vi "H5Pget_fill_value.vi"(4 "Data type":variant, 5 "HDF5 Type Ref (match data)":T1, 6 "error in (no error)":errorcluster, 9 "HDF5 Property Ref":T1) -> (0 "error out":errorcluster, 1 "Data Element":variant, 3 "HDF5 Ref out":T1)   [LabVIEW 2017]
doc: "Retrieves a dataset fill value."
uses:
  <vilib>/UPVI/lvhdf5/library.llb/HDF5 Ref.ctl
  <vilib>/UPVI/lvhdf5/identifier.llb/H5Iget_type.vi
  <vilib>/UPVI/lvhdf5/h5helper.dll
panel:
  # "LVHDF5 Toolkit\nCopyright (c) 2005-2013 by Jason D. Sommerville\nCopyright (c) 2014 by UPVI, LLC.\n\nThis use and distribution of this file is governed by the terms found in \nLICENSE.txt distributed with this toolkit and installed at\n <user.lib>\\_lvhdf5\\LICENSE.txt"
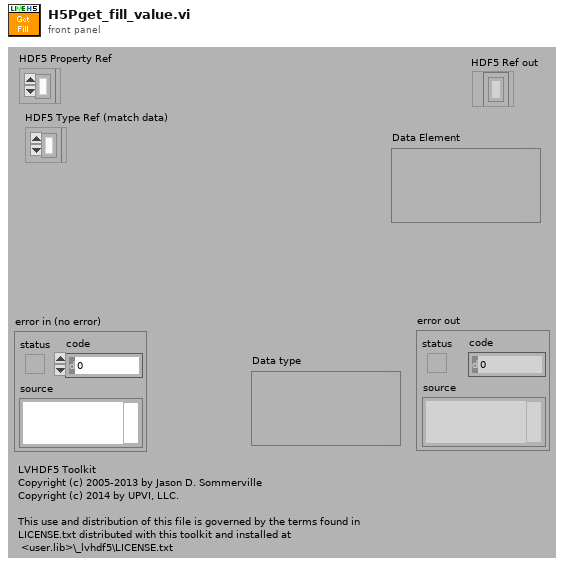
[diagram p1: front panel]
types:
  T1 = typedef "HDF5 Ref.ctl" = refnum<k1>
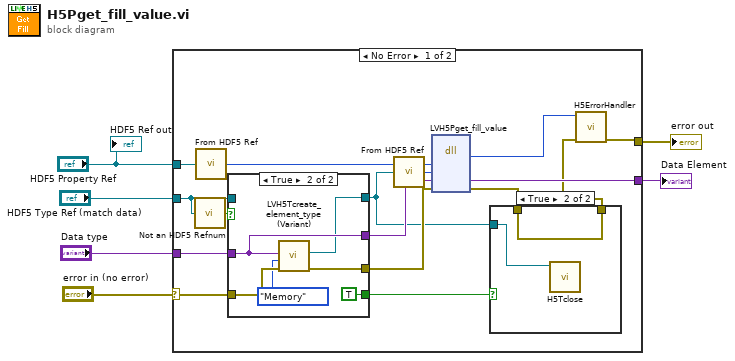
[diagram p0: block diagram]
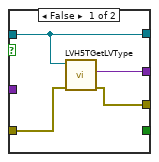
[diagram p3: hidden frame]
diagram:
  n1 = case shown="No Error" "error in (no error)" {
    selector: "error in (no error)" -> [w17 w36]
    tunnel: [w9 w36] -> w5
    tunnel: "HDF5 Property Ref" -> [w22 _]
    tunnel: "Data type" -> [w19 _]
    tunnel: "HDF5 Type Ref (match data)" -> [w18 _]
    tunnel: [w13 _] -> w1
    frame No Error {
      n2 = call <vilib>:"Not an HDF5 Refnum.vi"("HDF5 Ref"=w18) -> ("Not an HDF5 Refnum"=w20:bool)
      n3 = call <vilib>:"From HDF5 Ref.vi"("HDF5 Ref"=w22) -> ("I32"=w21:i32)
      n4 = case shown="True" w20 {
        tunnel: w19 -> [_ w33]
        tunnel: w18 -> [w29 _]
        tunnel: w17 -> [w27 w35]
        tunnel: [w29 w31] -> w11
        tunnel: [w28 w33] -> w16
        tunnel: [w26 w32] -> w15
        tunnel: [_ TRUE] -> w12
        frame False {
          n5 = call <vilib>:"LVH5TGetLVType.vi"("error in (no error)"=w27, "HDF5 Type Ref"=w29) -> ("error out"=w26:errorcluster, "Data Type"=w28:variant)  [unwired: 5 in, 3 out]
        }
        frame True {
          n6 = call <vilib>:"LVH5Tcreate_element_type (Variant).vi"("error in (no error)"=w35, "Type"=enum16{"File", "Memory"}."Memory", "Data"=w33) -> ("error out"=w32:errorcluster, "HDF5 Type Ref"=w31:T1)  [unwired: 4 in, 3 out]
        }
      }
      n7 = call <vilib>:"From HDF5 Ref.vi"("HDF5 Ref"=w11) -> ("I32"=w14:i32)
      n8 = dll-call lib="C:/Program Files/National Instruments/LabVIEW 2017/vi.lib/UPVI/lvhdf5/h5helper.dll" fn="LVH5Pget_fill_value"("plist_id"=w21, "type_id"=w14, "plvvar"=w16, "error"=w15) -> ("return type"=w7:i32, "plvvar"=w13:variant, "error"=w10:errorcluster)  [unwired: 5 in, 2 out]
      n9 = case shown="True" w12 {
        tunnel: w11 -> [_ w25]
        tunnel: [w23 w24] -> w8
        tunnel: w10 -> [w23 w24]
        frame False {
        }
        frame True {
          n10 = call <vilib>:"H5Tclose.vi"("HDF5 Datatype Ref"=w25) -> ()  [unwired: 8 in, 1 out]
        }
      }
      n11 = call <vilib>:"H5ErrorHandler.vi"("error in (no error)"=w8, "herr_t"=w7) -> ("error out"=w9:errorcluster)  [unwired: 3 in, 4 out]
    }
    frame Error {
    }
  }
  "error out" <- w5
  "Data Element" <- w1
  "HDF5 Ref out" <- "HDF5 Property Ref"
